vi "Check Serial Number.vi"(8 "error in (no error)":errorcluster, 10 "Serial ID":string, 11 "Application in":refnum<class "Application.lvclass">) -> (0 "error out":errorcluster, 2 "Material Type":string, 3 "Application out":refnum<class "Application.lvclass">, 5 "Gold Board":bool)   [LabVIEW 2017, in "Application.lvlib" / "Application.lvclass"]
doc: "Performs serial number and gold board lookup on a given LotID. If MES is enabled, it performs a material lookup using MES, if disabled it prompts the user."
uses:
  Application.lvclass
  Golden Board/Class/Golden Board.lvclass
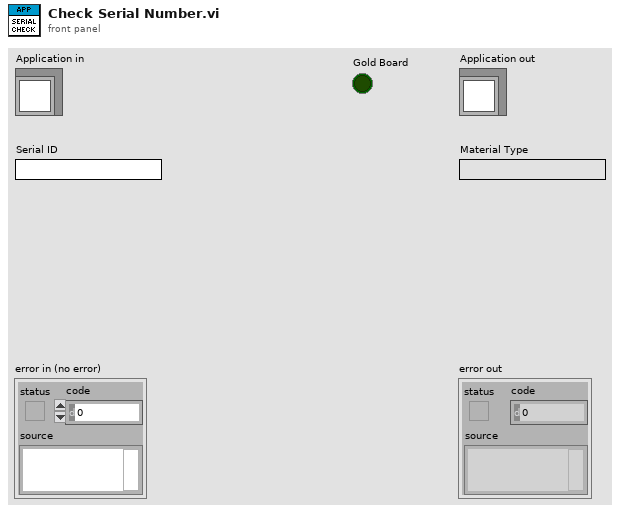
[diagram p1: front panel]
types:
  T1 = typedef "Application.lvlib/App Properties.lvclass/Class Properties -- Cluster.ctl" = cluster{"UUT Info":T2[], "Test Information":refnum<vi>, "Gold Board":refnum<class "Golden Board.lvclass">, "Test Recipe":refnum<class "Test Recipe.lvclass">, "Instruments":refnum<class "Instrument.lvclass">[], "Mode":T3, "Test Results":T4[], "Station Config":refnum<class "Station Config.lvclass">, "Variable Engine":refnum<class "Variable Engine.lvclass">}
  T2 = typedef "Application.lvlib/App Properties.lvclass/UUT Reference -- Cluster.ctl" = cluster{"Serial Number Reference":refnum<vi>, "Status Message Reference":refnum<vi>}
  T3 = typedef "Application.lvlib/Application.lvclass/Op Mode -- Enum.ctl" = u16
  T4 = typedef "Application.lvlib/App Properties.lvclass/Test Result -- Cluster.ctl" = cluster{"Position":i32, "Pass":bool, "Fail Codes":string}
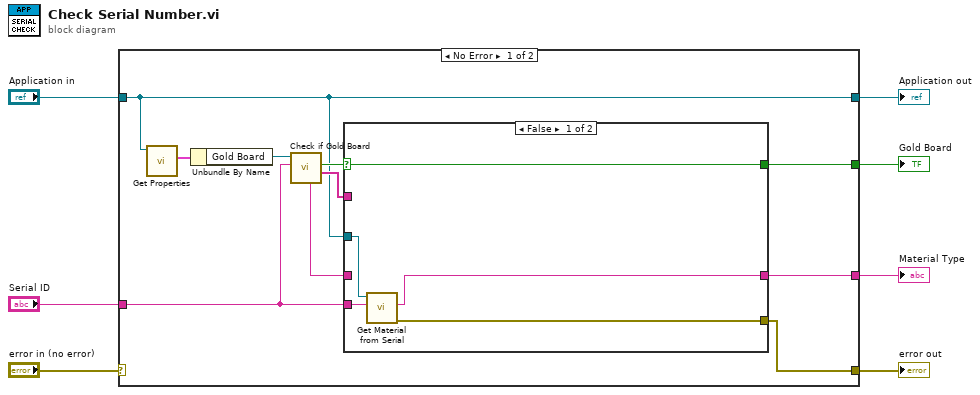
[diagram p0: block diagram]
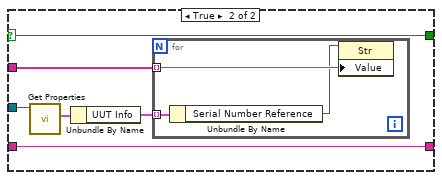
[diagram p2: hidden frame]
diagram:
  n1 = case shown="No Error" "error in (no error)" {
    selector: "error in (no error)" -> [_ w33]
    tunnel: [w9 w33] -> w6
    tunnel: [w8 w32] -> w4
    tunnel: "Application in" -> [w8 w32]
    tunnel: [w17 _] -> w3
    tunnel: [w10 _] -> w2
    tunnel: "Serial ID" -> [w16 _]
    frame No Error {
      n2 = call "Get Properties.vi"("Acrobat Template in"=w8) -> ("Class Properties"=w12:T1)  [unwired: 8 in, 2 out]
      n3 = Unbundle By Name(w12) -> ("Gold Board"=w11:refnum<class "Golden Board.lvclass">)
      n4 = call "Check if Gold Board.vi"("Serial Number"=w16, "Golden Board in"=w11) -> ("GoldSerNos"=w14:string[], "Gold Board"=w15:bool, "Material Name"=w13:string)  [unwired: 5 in, 2 out]
      n5 = case shown="False" w15 {
        selector: w15 -> [w18 w28]
        tunnel: [w18 w28] -> w17
        tunnel: [w20 _] -> w9
        tunnel: [w19 w27] -> w10
        tunnel: w8 -> [w22 w26]
        tunnel: w16 -> [w21 _]
        tunnel: w14 -> [_ w24]
        tunnel: w13 -> [_ w27]
        frame False {
          n6 = call-dynamic "Get Material from Serial.vi"("Serial ID"=w21, "Application in"=w22) -> ("error out"=w20:errorcluster, "Material Type"=w19:string)  [unwired: 7 in, 1 out]
        }
        frame True {
          n7 = call "Get Properties.vi"("Acrobat Template in"=w26) -> ("Class Properties"=w25:T1)  [unwired: 8 in, 2 out]
          n8 = Unbundle By Name(w25) -> ("UUT Info"=w23:T2[])
          n9 = for {
            tunnel: w24 -> [w31] mode=indexing
            tunnel: w23 -> [w30] mode=indexing
            n10 = Unbundle By Name(w30) -> ("Serial Number Reference"=w29:refnum<vi>)
            n11 = property class="Str"(reference=w29, "Value"=w31) -> ()  [unwired: 1 in, 2 out]
          }
        }
      }
    }
    frame Error {
    }
  }
  "error out" <- w6
  "Application out" <- w4
  "Gold Board" <- w3
  "Material Type" <- w2
